vi "test - Round Trip - Numeric - U32 Array.vi"(8 "error in (no error)":errorcluster, 11 "TestCase in":refnum<class "Python Data Tools Tests.lvclass">) -> (0 "error out":errorcluster, 3 "TestCase out":refnum<class "Python Data Tools Tests.lvclass">)   [LabVIEW 2013, in "Python Data Tools Tests.lvclass"]
uses:
  Python Data Tools Tests.lvclass
  <vilib>/addons/_JKI Toolkits/VI Tester/TestCase.llb/TestCase.lvclass
panel:
  out "Python String":string
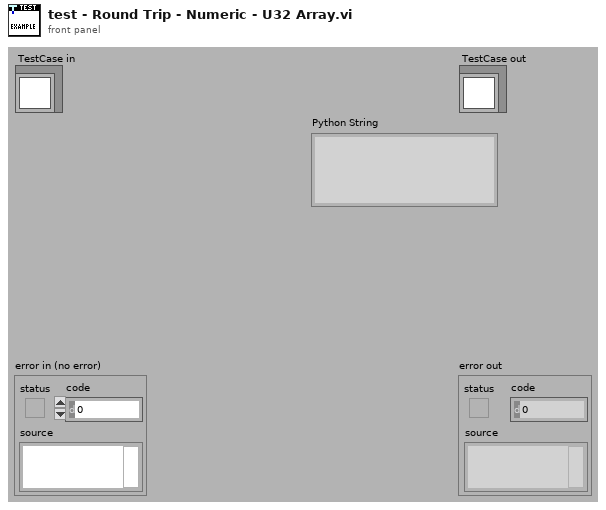
[diagram p1: front panel]
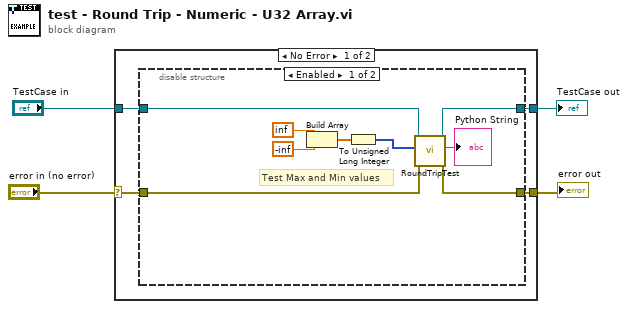
[diagram p0: block diagram]
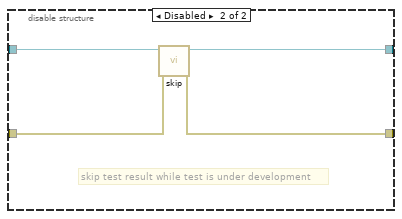
[diagram p2: hidden frame]
diagram:
  n1 = case shown="No Error" "error in (no error)" {
    selector: "error in (no error)" -> [w6 w23]
    tunnel: [w5 w23] -> w3
    tunnel: [w7 w22] -> w1
    tunnel: "TestCase in" -> [w8 w22]
    frame No Error {
      n2 = disable-structure shown="Enabled" {
        disable-tunnel: w8 -> [w17 w21]
        disable-tunnel: [w16 w18] -> w7
        disable-tunnel: w6 -> [w14 w20]
        disable-tunnel: [w15 w19] -> w5
        frame Enabled {
          # "Test Max and Min values"
          n3 = Build Array(inf, -inf) -> (w11:dbl[])
          n4 = To Unsigned Long Integer(number=w11) -> (unsigned 32bit integer=w10:u32[])
          n5 = call "RoundTripTest.vi"("error in (no error)"=w14, "Variant"=w10, "TestCase in"=w17) -> ("error out"=w15:errorcluster, "Python String"=→"Python String":string, "TestCase out"=w16:refnum<class "Python Data Tools Tests.lvclass">)  [unwired: 6 in]
        }
        frame Disabled {
          # "skip test result while test is under development"
          n6 = call <vilib>:"skip.vi"("error in (no error)"=w20, "TestCase in"=w21) -> ("error out"=w19:errorcluster, "TestCase out"=w18:refnum<class "Python Data Tools Tests.lvclass">)  [unwired: 8 in]
        }
      }
    }
    frame Error {
    }
  }
  "error out" <- w3
  "TestCase out" <- w1
